vi "Lab 9 Exercise 3c - Fake Data Acquisition.vi"() -> (11 "Temperature":dbl(slide) scale=0.0..100.0)   [LabVIEW 2023]
panel:
  in  "Temp Scale":bool
  # "Deg C"
  # "Deg F"
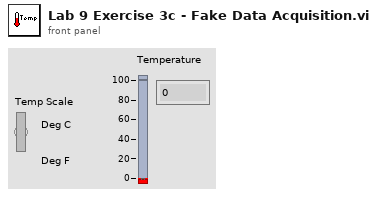
[diagram p1: front panel]
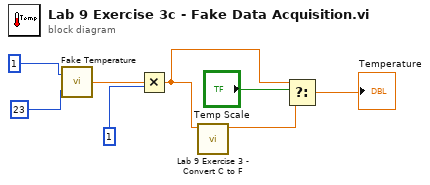
[diagram p0: block diagram]
diagram:
  n1 = call "Fake Temperature.vi"("Actual Temperature (C)"=23, "Temperature Noise"=1) -> ("Measured Temperature (C)"=w5:dbl)
  n2 = Multiply(x=w5, y=1) -> (x*y=w1:dbl)
  n3 = call "Lab 9 Exercise 3 - Convert C to F.vi"("deg C"=w1) -> ("deg F"=w2:dbl)  [unwired: 10 in]
  n4 = Select(t=w1, s="Temp Scale", f=w2) -> (s? t:f=→"Temperature":dbl)
